vi "OldWallFollow.vi"(3 "SupressIn":dbl, 7 "Inhibit":bool, 8 "HowAmI? Clean":cluster{"T":dbl, "Battery":dbl, "Temp":dbl}, 9 "WhatAroundMe? Clean":cluster{"T":dbl, "Range":dbl, "Bearing":dbl}[](array[cluster]), 10 "WhereAmI? Clean":T1, 11 "Velocity":dbl) -> (0 "SupressOut":dbl, 2 "ActCommand":dbl[](array[numeric]), 4 "InhibitOut":bool)   [LabVIEW 2010]
doc: "This subVI executes a wall folowing Midbrain behaviors. Its inputs are the outputs of the three SENSE processes, the overall velocity requested of the robot, a suppression value from another co-brahvior and an inhibit signal to turn the behavior off. The outputs are a 90 element steering array, a suppression value to diminish the output of co-behaviors and an inhibit output to shut off otehr behaviors.\n\nIt is designed to work with a 90 element behavior arbiter."
uses:
  <vilib>/addons/control/pid/pid.llb/PID (DBL).vi
  <vilib>/addons/control/pid/NI_PID_pid.lvlib
panel:
  # "This VI is a template for creating a robot subbehavior at the Midbrain level"
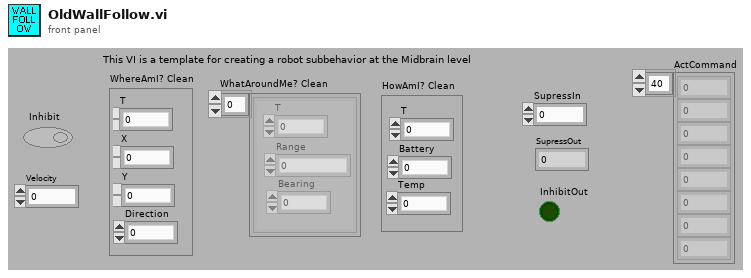
[diagram p1: front panel]
types:
  T1 = cluster{"T":dbl, "X":dbl, "Y":dbl, "Direction":dbl}
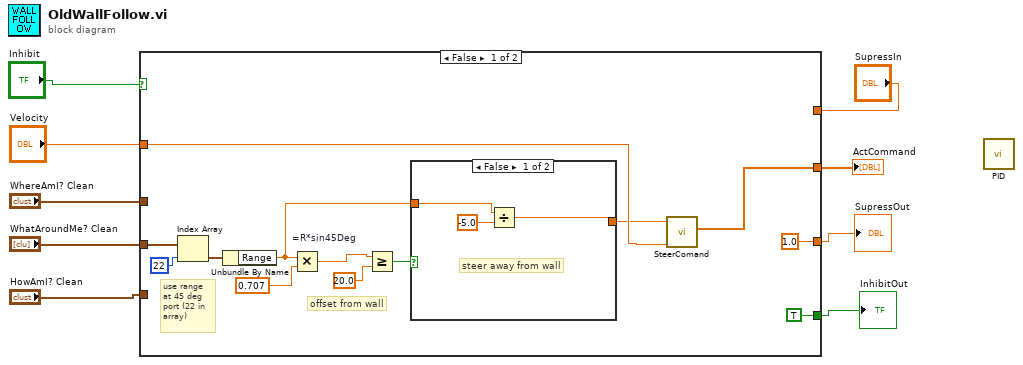
[diagram p0: block diagram]
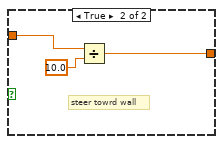
[diagram p2: hidden frame]
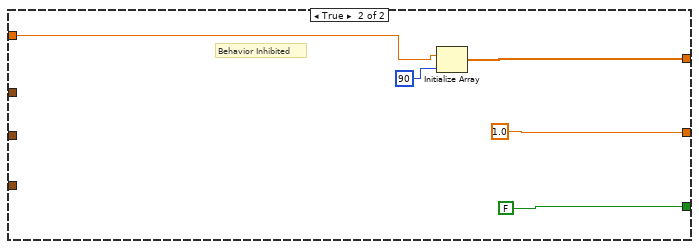
[diagram p3: hidden frame]
diagram:
  n1 = case shown="False" "Inhibit" {
    tunnel: "Velocity" -> [w14 w29]
    tunnel: "WhatAroundMe? Clean" -> [w20 _]
    tunnel: "WhereAmI? Clean" -> [_ _]
    tunnel: "HowAmI? Clean" -> [_ _]
    tunnel: "SupressIn" -> [_ _]
    tunnel: [w12 w31] -> w2
    tunnel: [1.0 ("SupressOut") 1.0 ("SupressOut")] -> w3
    tunnel: [TRUE ("InhibitOut") FALSE ("InhibitOut")] -> w1
    frame False {
      # "offset from wall"
      # "use range \nat 45 deg\nport (22 in\narray)"
      n2 = Index Array "Index Array"(array=w20, index=22) -> (element=w18:cluster{"T":dbl, "Range":dbl, "Bearing":dbl})
      n3 = Unbundle By Name(w18) -> ("Range"=w11:dbl)
      n4 = Multiply "=R*sin45Deg"(x=w11, y=0.707) -> (x*y=w16:dbl)
      n5 = Greater Or Equal?(x=w16, y=20.0) -> (x >= y?=w13:bool)
      n6 = case shown="False" w13 {
        tunnel: w11 -> [w25 w28]
        tunnel: [w23 w26] -> w10
        frame False {
          # "steer away from wall"
          n7 = Divide(x=w25, y=-5.0) -> (x/y=w23:dbl)
        }
        frame True {
          # "steer towrd wall"
          n8 = Divide(x=w28, y=10.0) -> (x/y=w26:dbl)
        }
      }
      n9 = call "SteerComand.vi"("Speed"=w14, "SteeringAngle"=w10) -> ("ManualActCommand"=w12:dbl[])  [unwired: 9 in]
    }
    frame True {
      # "Behavior Inhibited"
      n10 = Initialize Array "Initialize Array"(w29, 90 ("dimension size")) -> (w31:dbl[])
    }
  }
  "ActCommand" <- w2
  "SupressOut" <- w3
  "InhibitOut" <- w1
  n11 = call-poly <vilib>:"PID.vi"() -> ()  [unwired: 10 in, 2 out]
